vi "digital_out4.vi"() -> ()   [LabVIEW 2014]
doc: "Digital input output"
uses:
  <vilib>/DAQmx/write.llb/DAQmx Write (Digital 2D Bool NChan 1Samp NLine).vi
  <vilib>/DAQmx/create/channels.llb/DAQmx Create Channel (DO-Digital Output).vi
  <vilib>/DAQmx/miscellaneous.llb/DAQmx Fill In Error Info.vi
panel:
  in  "esci":bool
  in  "CONTROLLO LINEE":bool[][](array[boolean])=[[FALSE, FALSE, FALSE, TRUE]]
  in  "Scelta linee":tag="Dev1/port0/line3:0"
  # "Le linee 0,1,2,3 corrispondono ai\ncanali CB 52, 17, 49, 47"
  # "VERO"
  # "FALSO"
  # "47  49  17  52"
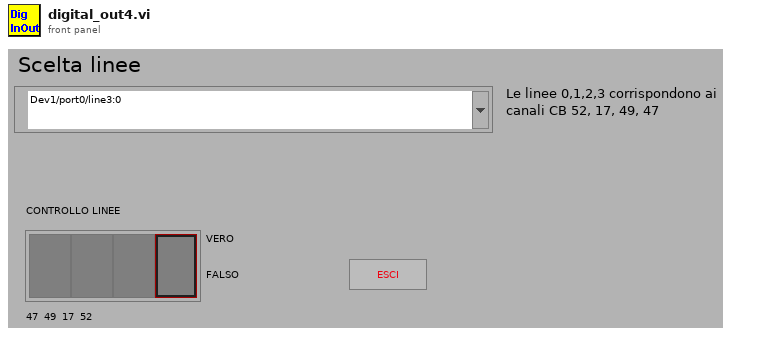
[diagram p1: front panel]
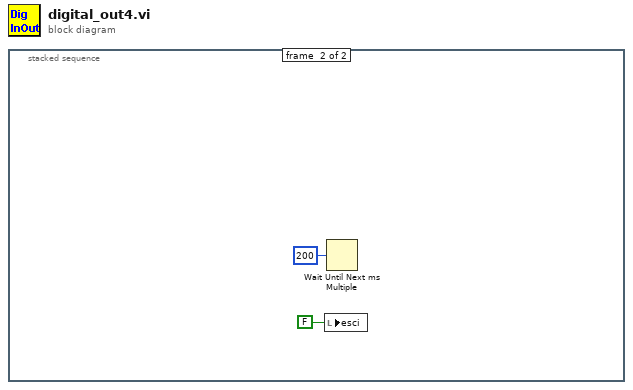
[diagram p0: block diagram]
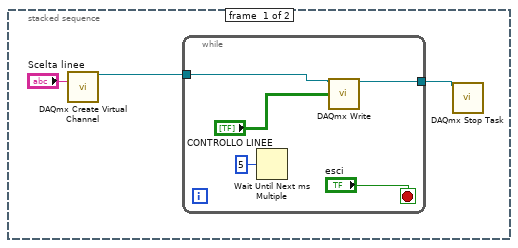
[diagram p2: hidden frame]
diagram:
  n1 = stacked-sequence {
    frame #0 {
      n2 = call-poly <vilib>:"DAQmx Create Virtual Channel.vi"("lines"="Scelta linee") -> ("task out"=w1:refnum<k21>)  [unwired: 13 in, 1 out]
      n3 = while {
        tunnel: [w8] -> w2
        tunnel: w1 -> [w7]
        stop <- "esci" stop-if-true
        n4 = Wait Until Next ms Multiple(millisecond multiple=u32 5) -> ()  [unwired: 1 out]
        n5 = call-poly <vilib>:"DAQmx Write.vi"("task/channels in"=w7, "data"="CONTROLLO LINEE") -> ("task out"=w8:refnum<k21>)  [unwired: 11 in, 2 out]
      }
      n6 = call <vilib>:"DAQmx Stop Task.vi"("task/channels in"=w2) -> ()  [unwired: 13 in, 2 out]
    }
    frame #1 {
      n7 = local write "esci"(FALSE ("esci")) -> ()
      n8 = Wait Until Next ms Multiple(millisecond multiple=u32 200) -> ()  [unwired: 1 out]
    }
  }
